vi "get_humidity.vi"(8 "error in (no error)":errorcluster, 11 "LightSourceMH110124MaiTai in":refnum<class "LightSourceMH110124MaiTai.lvclass">) -> (0 "error out":errorcluster, 2 "humidity":dbl, 3 "LightSourceMH110124MaiTai out":refnum<class "LightSourceMH110124MaiTai.lvclass">)   [LabVIEW 2010, in "LightSourceMH110124MaiTai.lvclass"]
uses:
  LightSourceMH110124MaiTai.lvclass
  LightSourceMH110124MaiTai.lvclass/LightSourceMH110124MaiTai.ctl
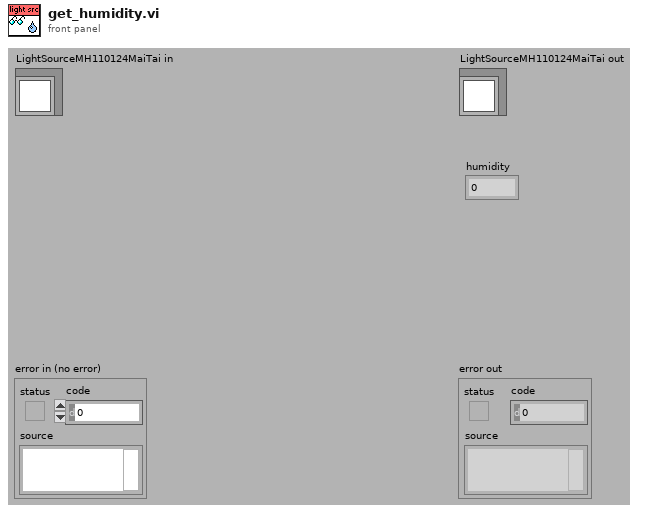
[diagram p1: front panel]
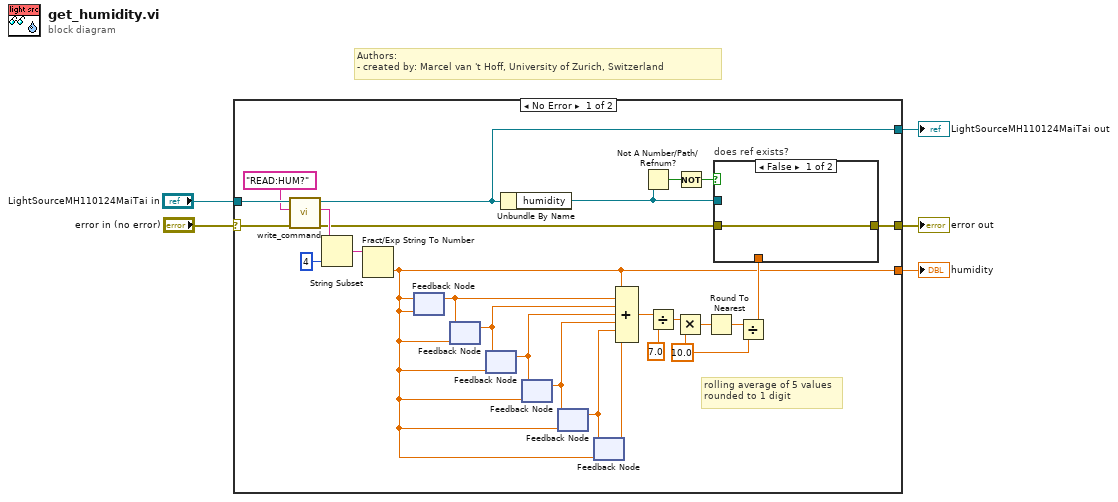
[diagram p0: block diagram]
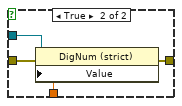
[diagram p2: hidden frame]
diagram:
  # "Authors: \n- created by: Marcel van 't Hoff, University of Zurich, Switzerland"
  n1 = case shown="No Error" "error in (no error)" {
    selector: "error in (no error)" -> [w30 w38]
    tunnel: [w23 w38] -> w3
    tunnel: [w25 w37] -> w2
    tunnel: "LightSourceMH110124MaiTai in" -> [w31 w37]
    tunnel: [w8 _] -> w1
    frame No Error {
      w19 = 10.0 ("y")
      # "rolling average of 5 values\nrounded to 1 digit"
      n2 = call-dynamic "write_command.vi"("error in (no error)"=w30, "string to write"="READ:HUM?", "LightSourceMH110124MaiTai in"=w31) -> ("error out"=w24:errorcluster, "read string"=w28:string, "LightSourceMH110124MaiTai out"=w25:refnum<class "LightSourceMH110124MaiTai.lvclass">)  [unwired: 6 in]
      n3 = String Subset(string=w28, length (rest)=4 ("length (rest)")) -> (substring=w27:string)  [unwired: 1 in]
      n4 = Fract/Exp String To Number(string=w27) -> (number=w8:dbl)  [unwired: 3 in, 1 out]
      n5 = feedback-in #1(w8) -> ()
      n6 = feedback #1(w8) -> (w22:dbl)
      n7 = feedback #2(w8) -> (w14:dbl)
      n8 = feedback-in #2(w22) -> ()
      n9 = feedback #3(w8) -> (w13:dbl)
      n10 = feedback-in #3(w14) -> ()
      n11 = Unbundle By Name(w25) -> ("humidity"=w12:refnum<vi>)
      n12 = feedback #4(w8) -> (w9:dbl)
      n13 = feedback-in #4(w13) -> ()
      n14 = feedback #5(w8) -> (w7:dbl)
      n15 = feedback-in #5(w9) -> ()
      n16 = feedback #6(w8) -> (w6:dbl)
      n17 = feedback-in #6(w7) -> ()
      n18 = Compound Arithmetic op=ADD(w8, w22, w14, w13, w9, w7, w6) -> (w21:dbl)
      n19 = Not A Number/Path/Refnum?(number/path/refnum=w12) -> (NaN/Path/Refnum?=w11:bool)
      n20 = Divide(x=w21, y=7.0) -> (x/y=w16:dbl)
      n21 = Multiply(x=w16, y=w19) -> (x*y=w17:dbl)
      n22 = Not(x=w11) -> (.not. x?=w10:bool)
      n23 = Round To Nearest(number=w17) -> (nearest integer value=w18:dbl)
      n24 = Divide(x=w18, y=w19) -> (x/y=w15:dbl)
      n25 = case "does ref exists?" shown="False" w10 {
        tunnel: w24 -> [w32 w36]
        tunnel: [w32 w35] -> w23
        tunnel: w15 -> [_ w34]
        tunnel: w12 -> [_ w33]
        frame False {
        }
        frame True {
          n26 = property class="DigNum (strict)"(reference=w33, error in=w36, "Value"=w34) -> (error out=w35:errorcluster)  [unwired: 1 out]
        }
      }
    }
    frame Error {
    }
  }
  "error out" <- w3
  "LightSourceMH110124MaiTai out" <- w2
  "humidity" <- w1
